vi "GSP_COLL_Global.vi"() -> ()   [LabVIEW 2015]
uses:
  SystemUtil/MotorStates.ctl
  SystemUtil/ThreadStates.ctl
panel:
  in  "Coll Thread State":T1
  in  "Coll Motor State":T2
  in  "COLL CPU Temp":dbl
  out "Coll Online":bool
  in  "Position":i32
  in  "Target":i32
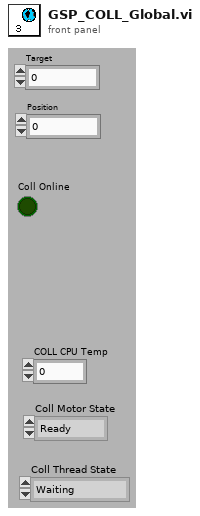
[diagram p1: front panel]
types:
  T1 = typedef "ThreadStates.ctl" = enum16{"Waiting", "Scripting", "Uninitialized", "Error"}
  T2 = typedef "MotorStates.ctl" = enum16{"Ready", "Moving", "Uninitialized", "Error"}
diagram:
